vi "Configure Voltage Measurement (Range).vi"(5 "Auto Voltage Range Upper Limit (20 V)":dbl=20.0, 6 "Auto Voltage Range Lower Limit (2 V)":dbl=2.0, 7 "Auto Voltage Range (T: Enable)":bool=TRUE, 8 "error in (no error)":errorcluster, 9 "Voltage Range (20 V)":dbl=20.0, 10 "Channel (1: Channel 1)":i32(ring)=1 items=["Channel 1"=1, "Channel 2"=2], 11 "VISA resource name":refnum<visa-resource-name>) -> (0 "error out":errorcluster, 3 "VISA resource name out":refnum<visa-resource-name>)   [LabVIEW 2012, in "Keysight B2980 Series.lvlib"]
doc: "Configures the range settings for voltage measurement function.\n\n<b>Note(s):</b>\n(1) This VI is only applicable for model B2985A and B2987A.\n(2) Voltage measurement should be enabled from <b>Configure Measurement Function.vi</b>."
uses:
  Keysight B2980 Series.lvlib
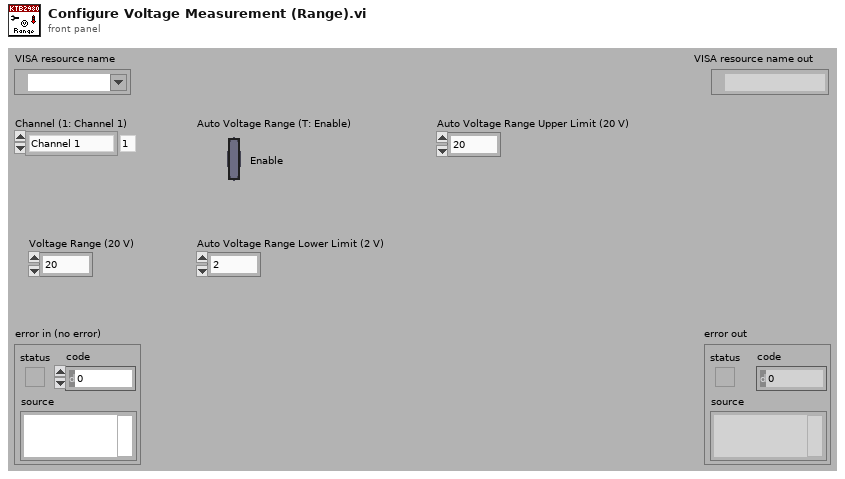
[diagram p1: front panel]
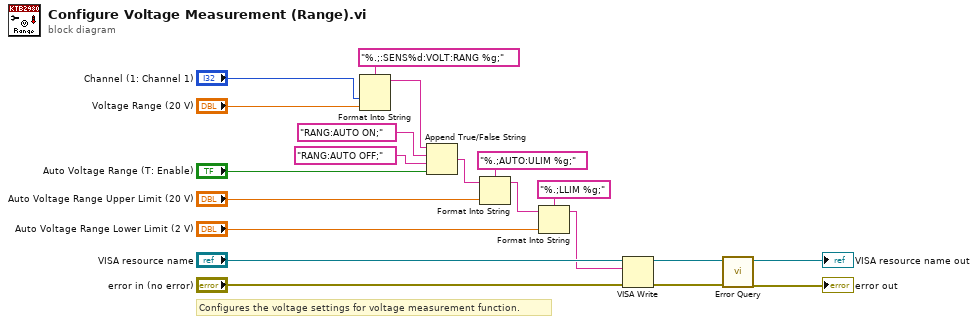
[diagram p0: block diagram]
diagram:
  # "Configures the voltage settings for voltage measurement function."
  n1 = Format Into String(format string="%.;:SENS%d:VOLT:RANG %g;", "Channel (1: Channel 1)", "Voltage Range (20 V)") -> (resulting string=w11:string)  [unwired: 2 in, 1 out]
  n2 = Append True/False String(1:"Auto Voltage Range (T: Enable)", 2:"RANG:AUTO OFF;", 3:"RANG:AUTO ON;", 4:w11) -> (0:w9:string)
  n3 = Format Into String(format string="%.;AUTO:ULIM %g;", initial string=w9, "Auto Voltage Range Upper Limit (20 V)") -> (resulting string=w7:string)  [unwired: 1 in, 1 out]
  n4 = Format Into String(format string="%.;LLIM %g;", initial string=w7, "Auto Voltage Range Lower Limit (2 V)") -> (resulting string=w6:string)  [unwired: 1 in, 1 out]
  n5 = VISA Write(VISA resource name="VISA resource name", write buffer=w6, error in (no error)="error in (no error)") -> (VISA resource name out=w18:refnum<visa-resource-name>, error out=w17:errorcluster)  [unwired: 1 out]
  n6 = call "Error Query.vi"("error in (no error)"=w17, "VISA resource name"=w18) -> ("error out"=→"error out":errorcluster, "VISA resource name out"=→"VISA resource name out":refnum<visa-resource-name>)  [unwired: 8 out]
